vi "VL53L0X_SetVcselPulsePeriodFinalRange.vi"(6 "val":i32, 9 "addr":i32, 10 "?":T1, 11 "error in (no error)":errorcluster) -> (2 "Status":bool, 3 "error out":errorcluster)   [LabVIEW 2019, in "DistanceSensorDriver.lvlib"]
uses:
  DistanceSensorDriver.lvlib
  Typedef/Ports.ctl
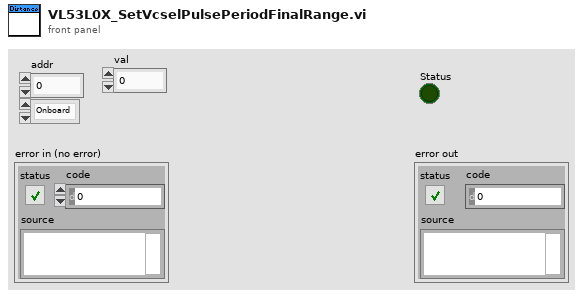
[diagram p1: front panel]
types:
  T1 = typedef "DistanceSensorDriver.lvlib/Ports.ctl" = enum32{"Onboard", "MXP"}
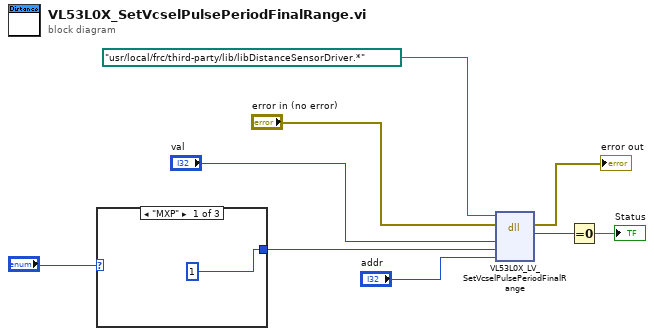
[diagram p0: block diagram]
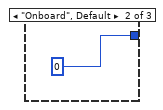
[diagram p2: hidden frame]
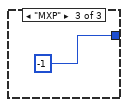
[diagram p3: hidden frame]
diagram:
  n1 = case shown="\"MXP\"" "?" {
    tunnel: [1 ("port") 0 ("port") -1 ("port")] -> w6
    frame "MXP" {
    }
    frame "Onboard", Default {
    }
    frame "MXP" {
    }
  }
  n2 = dll-call lib="?" fn="VL53L0X_LV_SetVcselPulsePeriodFinalRange"(path in=path "/usr/local/frc/third-party/lib/libDistanceSensorDriver.*", error in="error in (no error)", "val"="val", "port"=w6, "addr"="addr") -> (error out=→"error out":errorcluster, "return type"=w5:i32)  [unwired: 4 in, 1 out]
  n3 = Equal To 0?(x=w5) -> (x = 0?=→"Status":bool)
